vi "main.vi"() -> ()   [LabVIEW 2021]
uses:
  Peasant/PeasantCluster.ctl
  Peasant/Peasant.lvclass
  Knight/Knight.lvclass
  W:/School/AnimoProgramovani2/2024/Arena/Peasant/Peasant.lvclass
  Peasant/Peasant.lvclass/Peasant.ctl
  Peasant/Read Peasant Attributes.vi
  Peasant/Write Peasant Attributes.vi
panel:
  in  "Reinit1":bool
  out "error out":errorcluster
  out "Cube 2":i32
  out "Cube 1":i32
  in  "Attack 2":bool
  in  "Attack 1":bool
  in  "Stop":bool
  out "Peasant 2":T1
  out "Peasant 1":T1
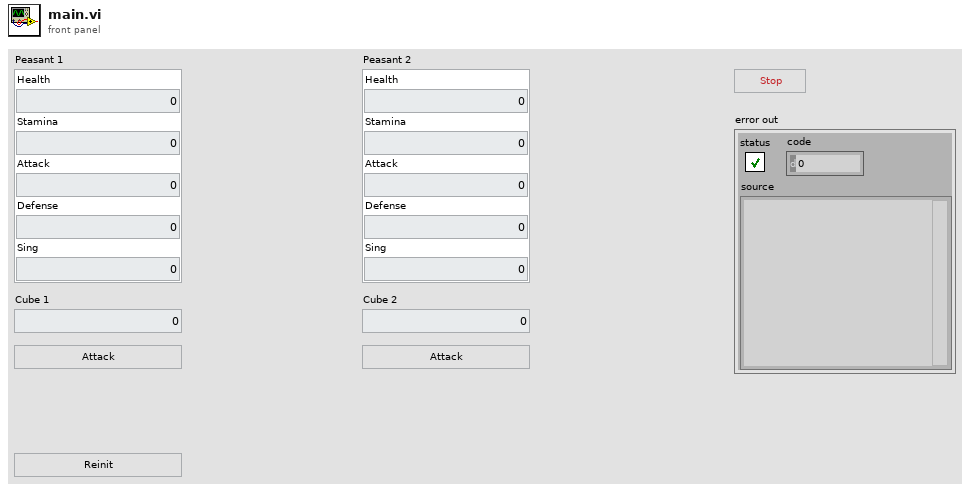
[diagram p1: front panel]
types:
  T1 = typedef "PeasantCluster.ctl" = cluster{"Health":i32, "Stamina":i32, "Attack":i32, "Defense":i32, "Sing":i32}
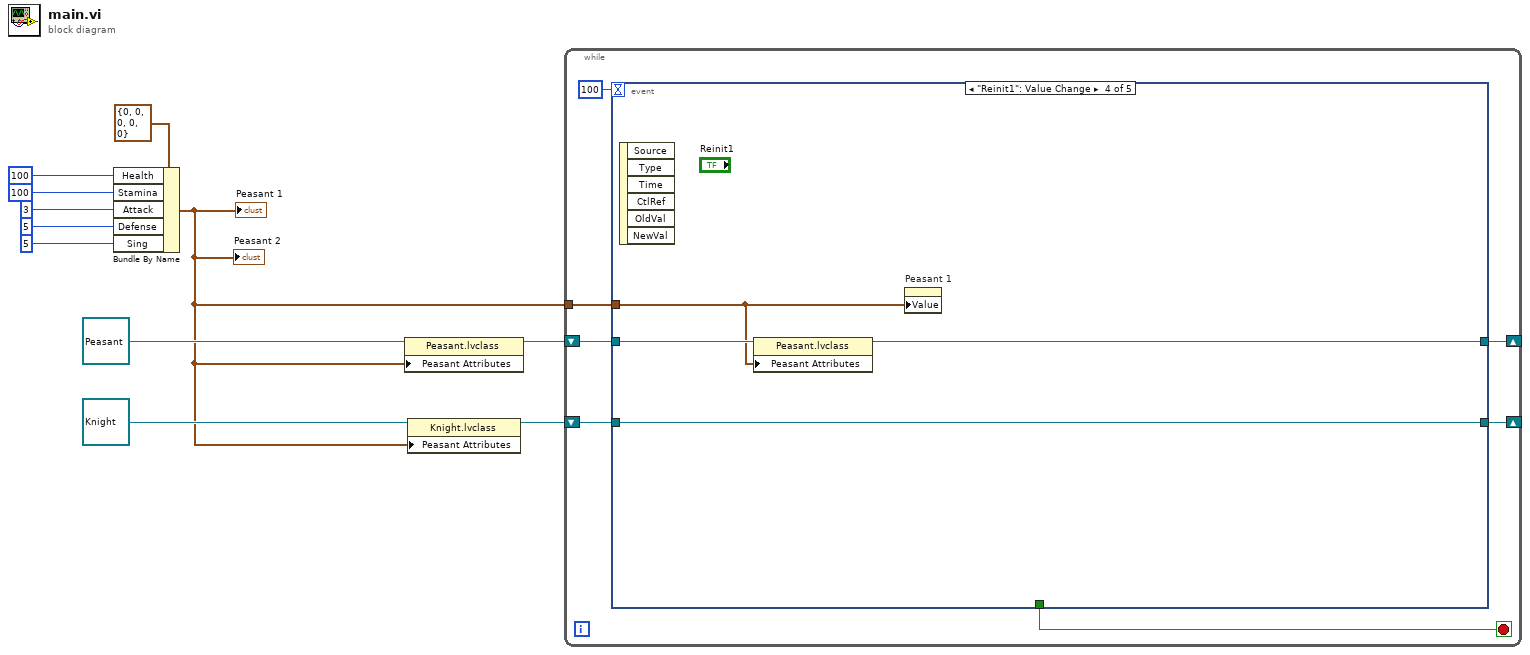
[diagram p0: block diagram]
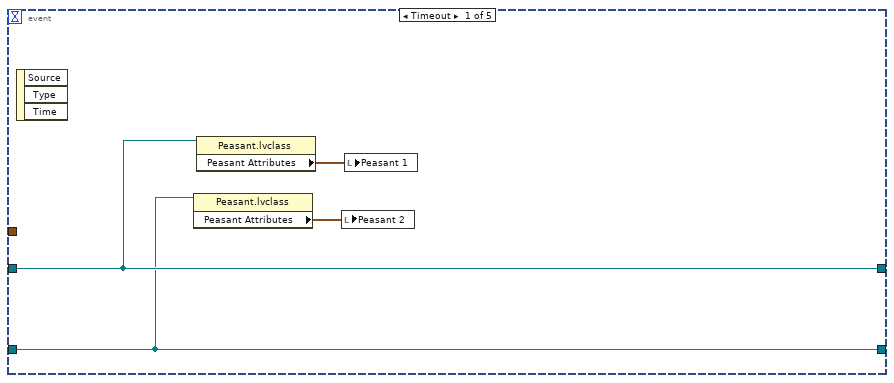
[diagram p2: hidden frame]
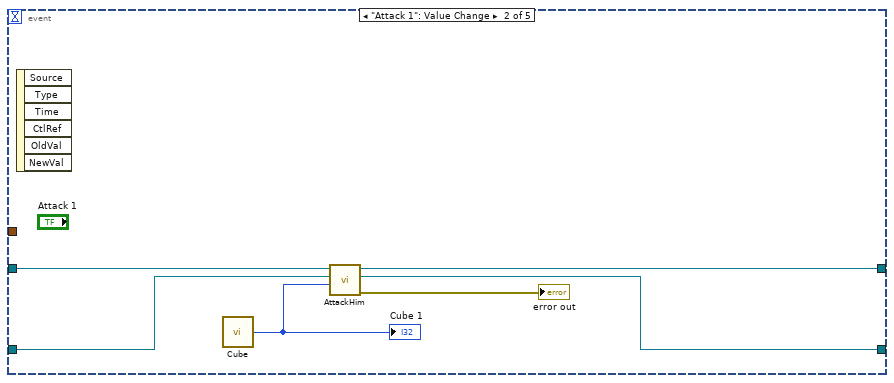
[diagram p3: hidden frame]
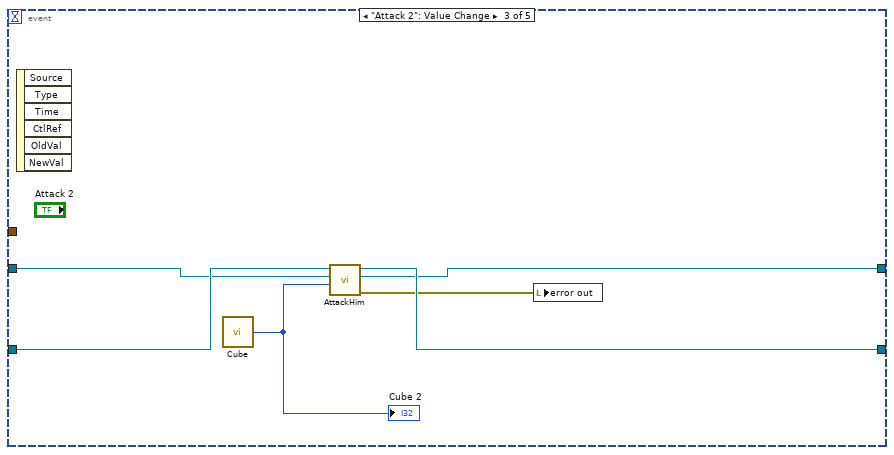
[diagram p4: hidden frame]
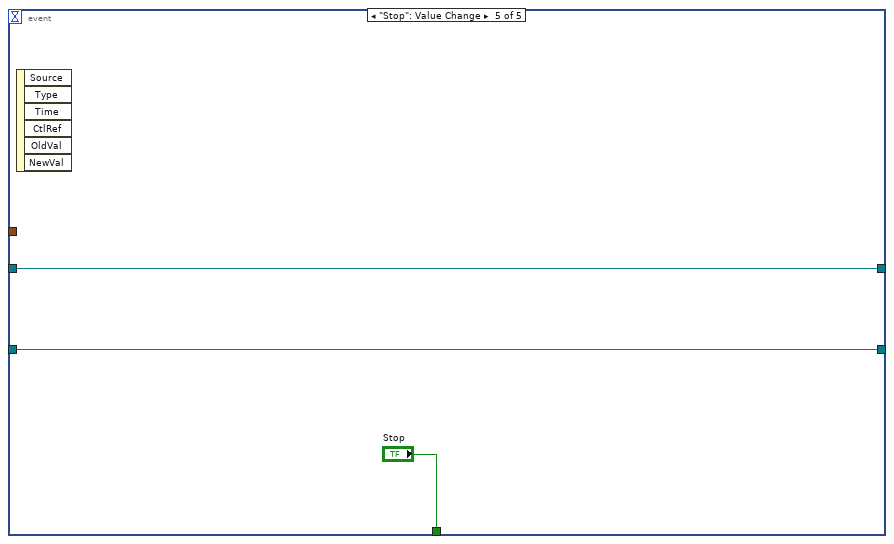
[diagram p5: hidden frame]
diagram:
  n1 = Bundle By Name(cluster=T1 {"Health"=0, "Stamina"=0, "Attack"=0, "Defense"=0, "Sing"=0} ("Peasant 1"), "Health"=100, "Stamina"=100, "Attack"=3, "Defense"=5, "Sing"=5) -> (w1:T1)
  "Peasant 1" <- w1
  "Peasant 2" <- w1
  n2 = property class="Peasant.lvclass"(reference=refnum<class "Peasant.lvclass"> refnum ("Peasant.lvclass"), "Peasant Attributes"=w1) -> (reference out=w5:refnum<class "Peasant.lvclass">)  [unwired: 1 in, 1 out]
  n3 = property class="Knight.lvclass"(reference=refnum<class "Knight.lvclass"> refnum ("Knight.lvclass"), "Peasant Attributes"=w1) -> (reference out=w4:refnum<class "Knight.lvclass">)  [unwired: 1 in, 1 out]
  n4 = while {
    shift-right: [w14] -> _
    shift-left: w5 -> [w15]
    shift-right: [w16] -> _
    shift-left: w4 -> [w17]
    tunnel: w1 -> [w12]
    stop <- w18 stop-if-true
    n5 = event shown="[3] \"Reinit1\": Value Change" {
      selector: _ -> [_ _ _ _ _]
      dyn-events: _ -> [_ _ _ _ _]
      timeout: 100 -> [_ _ _ _ _]
      tunnel: [_ _ _ _ "Stop"] -> w18
      tunnel: w17 -> [w20 w27 w34 w35 w40]
      tunnel: [w20 w25 w32 w35 w40] -> w16
      tunnel: w15 -> [w22 w28 w33 w38 w39]
      tunnel: [w22 w26 w31 w37 w39] -> w14
      tunnel: w12 -> [_ _ _ w36 _]
      event Timeout {
        n6 = event-data() -> ()  [unwired: 1 in, 3 out]
        n7 = property class="Peasant.lvclass"(reference=w20) -> ("Peasant Attributes"=w19:T1)  [unwired: 1 in, 2 out]
        n8 = property class="Peasant.lvclass"(reference=w22) -> ("Peasant Attributes"=w21:T1)  [unwired: 1 in, 2 out]
        n9 = local write "Peasant 2"(w19) -> ()
        n10 = local write "Peasant 1"(w21) -> ()
      }
      event "Attack 1": Value Change {
        n11 = event-data() -> ()  [unwired: 1 in, 6 out]
        n12 = call "Cube.vi"() -> ("Number"=w24:u64)
        "Cube 1" <- w24
        n13 = call-dynamic "AttackHim.vi"("Cube"=w24, "Rival"=w27, "Peasant in"=w28) -> ("error out"=→"error out":errorcluster, "Rival out"=w25:refnum<class "Peasant.lvclass">, "Peasant out"=w26:refnum<class "Peasant.lvclass">)  [unwired: 5 in, 1 out]
      }
      event "Attack 2": Value Change {
        n14 = event-data() -> ()  [unwired: 1 in, 6 out]
        n15 = call "Cube.vi"() -> ("Number"=w30:u64)
        "Cube 2" <- w30
        n16 = call-dynamic "AttackHim.vi"("Cube"=w30, "Rival"=w33, "Peasant in"=w34) -> ("error out"=w29:errorcluster, "Rival out"=w31:refnum<class "Peasant.lvclass">, "Peasant out"=w32:refnum<class "Peasant.lvclass">)  [unwired: 5 in, 1 out]
        n17 = local write "error out"(w29) -> ()
      }
      event "Reinit1": Value Change {
        n18 = event-data() -> ()  [unwired: 1 in, 6 out]
        n19 = property class="Peasant.lvclass"(reference=w38, "Peasant Attributes"=w36) -> (reference out=w37:refnum<class "Peasant.lvclass">)  [unwired: 1 in, 1 out]
        n20 = property on="Peasant 1" class="Clust (strict)"("Value"=w36) -> ()  [unwired: 2 in, 2 out]
      }
      event "Stop": Value Change {
        n21 = event-data() -> ()  [unwired: 1 in, 6 out]
      }
    }
  }
